vi "Main (DAQ, 2 Task, Tag).vi"() -> ()   [LabVIEW 2018]
doc: "Datenerfassung - Producer/Consumer mit Zustandsmaschine und Tag Channel\n\n* Analoges Eingangssigna, Definition des\nDAQmx Kanals im NI Max\n* Realisierung mit eine Zustandsmaschine\n* Drei Schleifen (Tasks): Zustandsmaschine und Datenerfassung und Auswertung\n*Realisierung des User Interfaces mit Event Structure\n* Kommunikation benutzereingaben (Zustandsmaschine) zu Datenerfassung mit \"Tag Channel\" und \"Stream Channel\"\n* Anzeige der Events\n* Anzeige der Zustände \"Messung/Warten/Auswertung\""
uses:
  Type Definitions/States UI.ctl
  Type Definitions/States Worker.ctl
  <vilib>/DAQmx/read.llb/DAQmx Read (Analog Wfm 1Chan NSamp).vi
  <extravilib>/ChannelInstances/Tag-t'States Worker.ctl'/Read With Abort.vi
  <extravilib>/ChannelInstances/Tag-t'States Worker.ctl'/Write With Abort.vi
  <extravilib>/ChannelInstances/Tag-t'States Worker.ctl'/Instantiate.vi
  <extravilib>/ChannelInstances/Tag-t'States Worker.ctl'/EndpointRead.vi
  <vilib>/DAQmx/miscellaneous.llb/DAQmx Fill In Error Info.vi
  <vilib>/Waveform/WDTOps.llb/WDT Append Waveforms DBL.vi
  <extravilib>/ChannelInstances/Tag-t'States Worker.ctl'/Endpoint.vi
  <extravilib>/ChannelInstances/Tag-t'States Worker.ctl'.lvlib
panel:
  in  "Tab Control":enum32{"Graph", "Chart"}(tab)=enum."Chart"
  out "Graph":waveform(dbl)(graph)
  out "Chart":waveform(dbl)(graph)
  out "Messung":bool
  out "Events":string="Exit= 1"
  in  "Messung":bool
  in  "Exit":bool
  out "Anzeige":dbl(knob) scale=0.0..10.0 scale format="%1.1f"
  # "Datenerfassung - \"UI/Worker\" mit Zustandsmaschine und Tag Channel\n\n* Analoges Eingangssignal, Definition des\nDAQmx Kanals im NI Max\n*  Realisierung mit zwei Zustandsmaschinen\n* Zustandsmaschine für UI Events und für Worker-Aufgabe\n* Zwei Schleifen (Tasks): UI und, Datenerfassung&Auswertung\n*Realisierung des User Interfaces mit Event Structure\n* Kommunikation Benutzereingaben (Zustandsmaschine) zu Datenerfassung mit \"Tag Channel\"\n\n* Anzeige der Events\n* Anzeige der Zustände \"Messung/Warten/Auswertung\"\n\nTiming\n* Task 1Khz Sampling Rate und 100 Samples\n* Gemessen jede 1sec (Timed loop)"
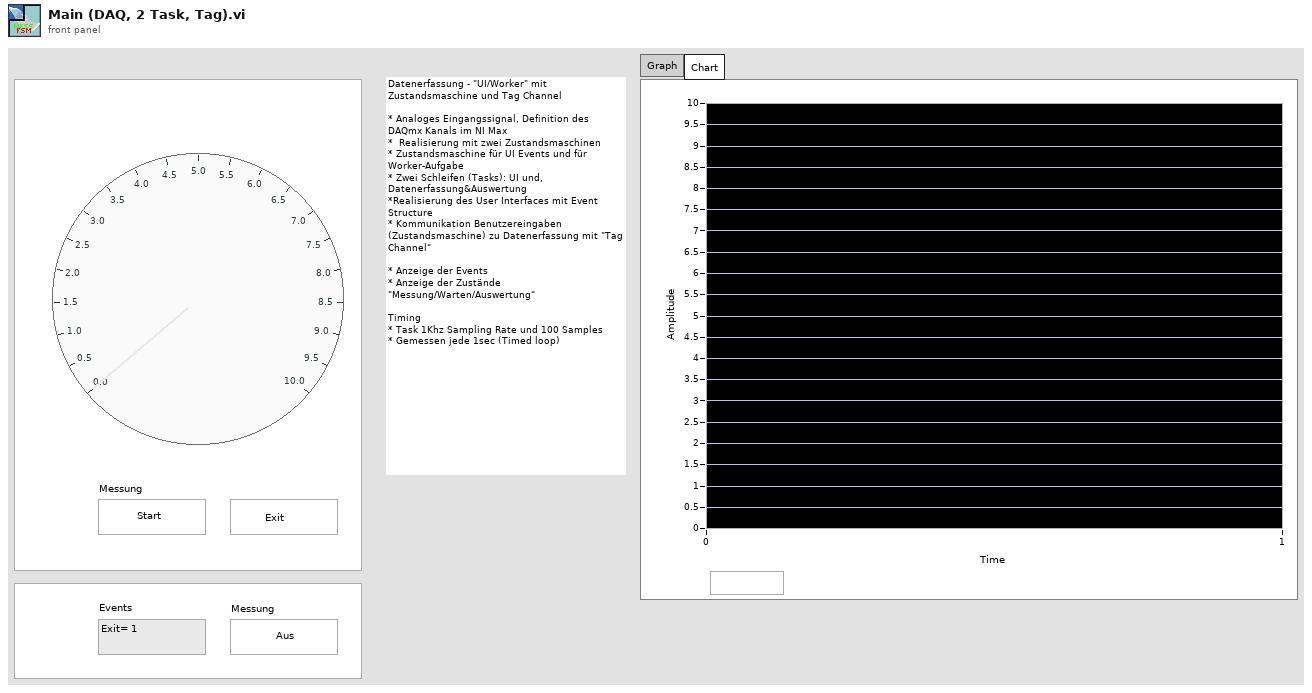
[diagram p1: front panel]
types:
  T1 = typedef "States UI.ctl" = enum16{"Initialize", "Wait for Event", "Exit"}
  T2 = typedef "States Worker.ctl" = enum16{"Messen", "Pausieren", "Exit"}
  T3 = typedef "Tag-t'States Worker.ctl'.lvlib/))Channel.ctl" = refnum<queue>
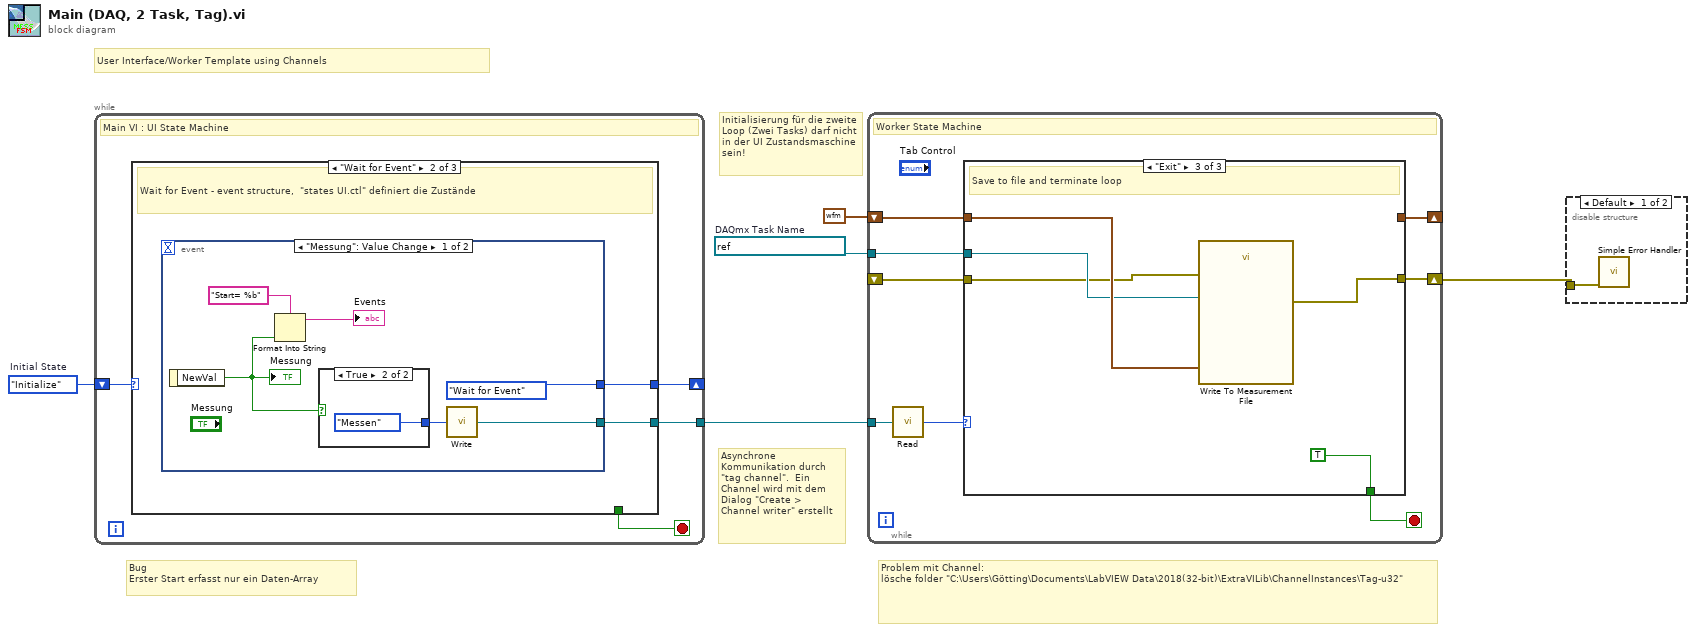
[diagram p0: block diagram]
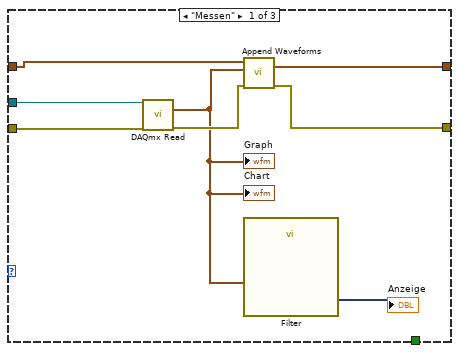
[diagram p2: hidden frame]
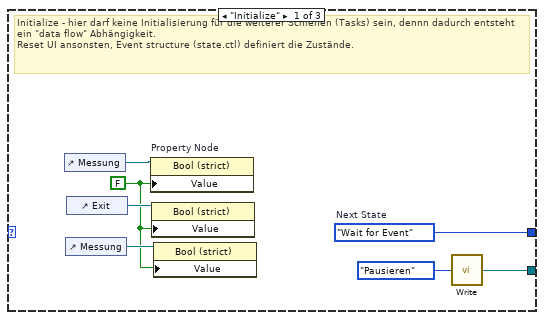
[diagram p4: hidden frame]
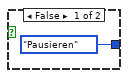
[diagram p5: hidden frame]
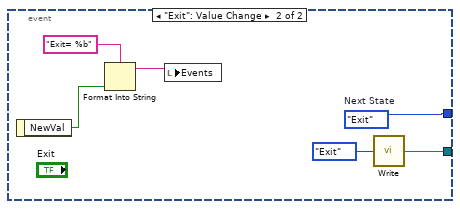
[diagram p6: hidden frame]
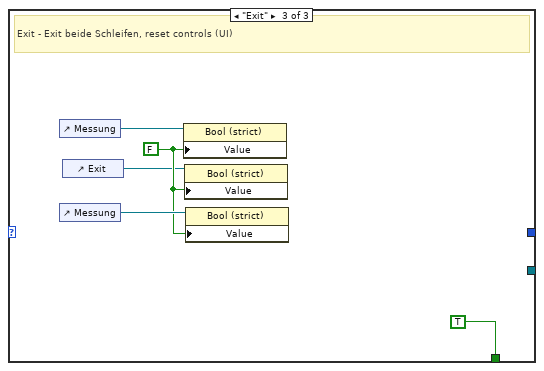
[diagram p7: hidden frame]
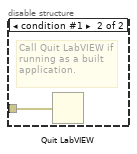
[diagram p8: hidden frame]
diagram:
  w4 = refnum<k21> "Spannung_1kHz100"  # DAQmx Task Name
  w5 = States_UI."Initialize"  # Initial State
  # "Bug\nErster Start erfasst nur ein Daten-Array"
  # "User Interface/Worker Template using Channels"
  # "Problem mit Channel:\nlösche folder \"C:\\Users\\Götting\\Documents\\LabVIEW Data\\2018(32-bit)\\ExtraVILib\\ChannelInstances\\Tag-u32\""
  # "Initialisierung für die zweite Loop (Zwei Tasks) darf nicht in der UI Zustandsmaschine sein!"
  # "Asynchrone Kommunikation durch\n\"tag channel\".  Ein Channel wird mit dem\nDialog \"Create > Channel writer\" erstellt"
  n1 = while {
    shift-right: [w8] -> _
    shift-left: w5 -> [w9]
    tunnel: [w6] -> w1
    stop <- w7 stop-if-true
    # "Main VI : UI State Machine"
    n2 = case shown="\"Wait for Event\"" w9 {
      tunnel: [w16 w18 _] -> w8
      tunnel: [_ _ TRUE ("Stop Loop?")] -> w7
      tunnel: [w10 w17 _] -> w6
      frame "Initialize" {
        w12 = FALSE ("Value")
        w16 = States_UI."Wait for Event"  # Next State
        # "Initialize - hier darf keine Initialisierung für die weiterer Schleifen (Tasks) sein, dennn dadurch entsteht ein \"data flow\" Abhängigkeit. \nReset UI ansonsten, Event structure (state.ctl) definiert die Zustände."
        n3 = control-ref of="Messung"() -> (w15:refnum<vi>)
        n4 = control-ref of="Messung"() -> (w13:refnum<vi>)
        n5 = control-ref of="Exit"() -> (w14:refnum<vi>)
        n6 = property on="Property Node" class="Bool (strict)"(reference=w15, "Value"=w12) -> ()  [unwired: 1 in, 2 out]
        n7 = property class="Bool (strict)"(reference=w14, "Value"=w12) -> ()  [unwired: 1 in, 2 out]
        n8 = property class="Bool (strict)"(reference=w13, "Value"=w12) -> ()  [unwired: 1 in, 2 out]
        n9 = call <extravilib>:"Write.vi"("element"=States_Worker."Pausieren" ("States")) -> ("channel"=w10:T3)  [unwired: 1 out]
      }
      frame "Wait for Event" {
        # "Wait for Event - event structure,  \"states UI.ctl\" definiert die Zustände"
        n10 = event shown="[0] \"Messung\": Value Change" {
          selector: _ -> [_ _]
          dyn-events: _ -> [_ _]
          timeout: _ -> [_ _]
          tunnel: [States_UI."Wait for Event" ("Next State") w32] -> w18
          tunnel: [w19 w27] -> w17
          event "Messung": Value Change {
            n11 = event-data() -> ("NewVal"=w21:bool)  [unwired: 1 in]
            "Messung" <- w21
            n12 = Format Into String(format string="Start= %b", w21) -> (resulting string=→"Events":string)  [unwired: 2 in, 1 out]
            n13 = case shown="True" w21 {
              tunnel: [States_Worker."Pausieren" ("Initial State") States_Worker."Messen" ("Initial State")] -> w20
              frame False {
              }
              frame True {
              }
            }
            n14 = call <extravilib>:"Write.vi"("element"=w20) -> ("channel"=w19:T3)  [unwired: 1 out]
          }
          event "Exit": Value Change {
            w32 = States_UI."Exit"  # Next State
            n15 = event-data() -> ("NewVal"=w30:bool)  [unwired: 1 in]
            n16 = Format Into String(format string="Exit= %b", w30) -> (resulting string=w31:string)  [unwired: 2 in, 1 out]
            n17 = local write "Events"(w31) -> ()
            n18 = call <extravilib>:"Write.vi"("element"=States_Worker."Exit" ("States")) -> ("channel"=w27:T3)  [unwired: 1 out]
          }
        }
      }
      frame "Exit" {
        w35 = FALSE ("Value")
        # "Exit - Exit beide Schleifen, reset controls (UI)"
        n19 = control-ref of="Messung"() -> (w37:refnum<vi>)
        n20 = control-ref of="Messung"() -> (w36:refnum<vi>)
        n21 = control-ref of="Exit"() -> (w34:refnum<vi>)
        n22 = property class="Bool (strict)"(reference=w37, "Value"=w35) -> ()  [unwired: 1 in, 2 out]
        n23 = property class="Bool (strict)"(reference=w34, "Value"=w35) -> ()  [unwired: 1 in, 2 out]
        n24 = property class="Bool (strict)"(reference=w36, "Value"=w35) -> ()  [unwired: 1 in, 2 out]
      }
    }
  }
  n25 = while {
    shift-right: [w45] -> w3
    shift-left: _ -> [w44]
    tunnel: w4 -> [w43]
    shift-right: [w41] -> _
    shift-left: waveform(dbl) {"t0"=timestamp(0 s since 1904-01-01), "dt"=1.0, "Y"=[]} ("Waveform") -> [w42]
    tunnel: w1 -> [w39]
    stop <- w40 stop-if-true
    # "Worker State Machine"
    n26 = call <extravilib>:"Read.vi"("channel"=w39) -> ("element"=w38:T2)  [unwired: 1 in, 1 out]
    n27 = case shown="\"Exit\"" w38 {
      tunnel: [w48 w54 w56] -> w45
      tunnel: w44 -> [w53 w54 w57]
      tunnel: w43 -> [w52 _ w58]
      tunnel: w42 -> [w50 w55 w59]
      tunnel: [w47 w55 _] -> w41
      tunnel: [_ _ TRUE ("abort")] -> w40
      frame "Messen" {
        n28 = call-poly <vilib>:"DAQmx Read.vi"("task/channels in"=w52, "error in"=w53) -> ("data"=w46:waveform(dbl), "error out"=w49:errorcluster)  [unwired: 11 in, 1 out]
        "Graph" <- w46
        "Chart" <- w46
        n29 = call-poly <vilib>:"Append Waveforms.vi"("error in (no error)"=w49, "waveform B"=w46, "waveform A"=w50) -> ("error out"=w48:errorcluster, "waveform out"=w47:waveform(dbl))  [unwired: 7 in]
        n30 = call "Filter"("Signal"=w46) -> ("Filtered Signal"=→"Anzeige":dynamicdata)  [unwired: 9 in, 1 out]
      }
      frame "Pausieren" {
        # "Do nothing, wait"
      }
      frame "Exit" {
        # "Save to file and terminate loop"
        n31 = call "Write To Measurement File"("Signals"=w59, "error in (no error)"=w57, "DAQmx Task"=w58) -> ("error out"=w56:errorcluster)  [unwired: 14 in, 2 out]
      }
    }
  }
  n32 = disable-structure shown="Default" {
    disable-tunnel: w3 -> [w61 w62]
    frame condition #0 (active) {
      n33 = call <vilib>:"Simple Error Handler.vi"("error in (no error)"=w61) -> ()  [unwired: 4 in, 5 out]
    }
    frame condition #1 {
      # "Call Quit LabVIEW if running as a built application."
      n34 = Quit LabVIEW(quit? (T)=w62) -> ()
    }
  }
